vi "Device Panel.vi"(7 "Calling VI Ref":refnum<vi>) -> ()   [LabVIEW 2020]
uses:
  Device Panel Controls/Device Control Information Array.ctl
  Device Panel Controls/Device Control Information.ctl
  <vilib>/Utility/miscctls.llb/LVPointTypeDef.ctl
  Device Manager/Common Device Queue/Common Device Controls/Common Device Actions.ctl
panel:
  in  "Quit All Engines":bool
  in  "Quit":bool
  in  "Devices":T1
  out "Hardware Configuration File Path":path
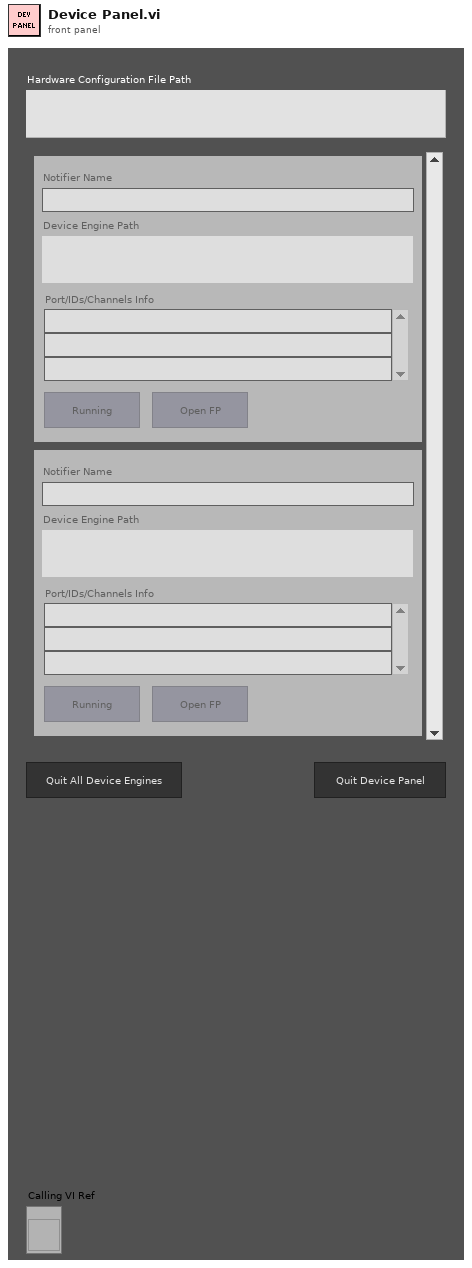
[diagram p1: front panel]
types:
  T1 = typedef "Device Control Information Array.ctl" = T2[]
  T2 = typedef "Device Control Information.ctl" = cluster{"Notifier Name":string, "Device Engine Path":path, "Running?":bool, "Open Front Panel":bool, "Port/IDs/Channels Info":string[]}
  T3 = enum16{"Always On", "Always Off", "Off While Running"}
  T4 = typedef "LVPointTypeDef.ctl" = cluster{"Horizontal":i16, "Vertical":i16}
  T5 = typedef "Common Device Actions.ctl" = enum16{"Specific Action", "Open Front Panel", "Close Front Panel", "Quit", "Quit All"}
  T6 = cluster{"Notifier Name":bool, "Device Engine Path":bool, "Running?":bool, "Open Front Panel":bool, "Port/IDs/Channels Info":bool[]}[]
  T7 = typedef "LVRectTypeDef.ctl" = cluster{"Left":i16, "Top":i16, "Right":i16, "Bottom":i16}
  T8 = typedef "LVBoundsTypeDef.ctl" = cluster{"Width":u32, "Height":u32}
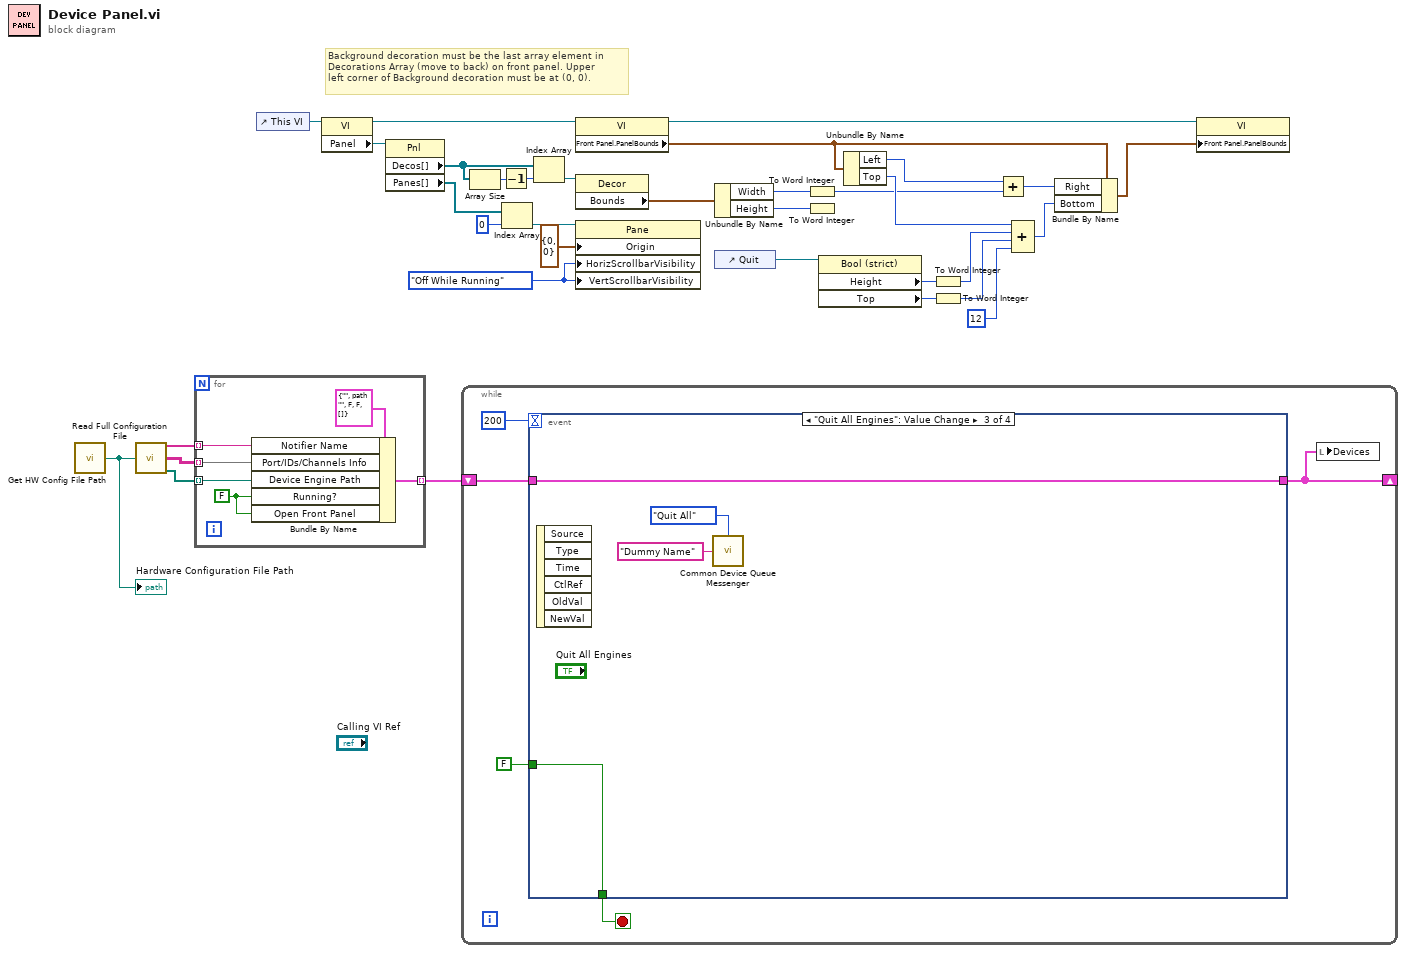
[diagram p0: block diagram]
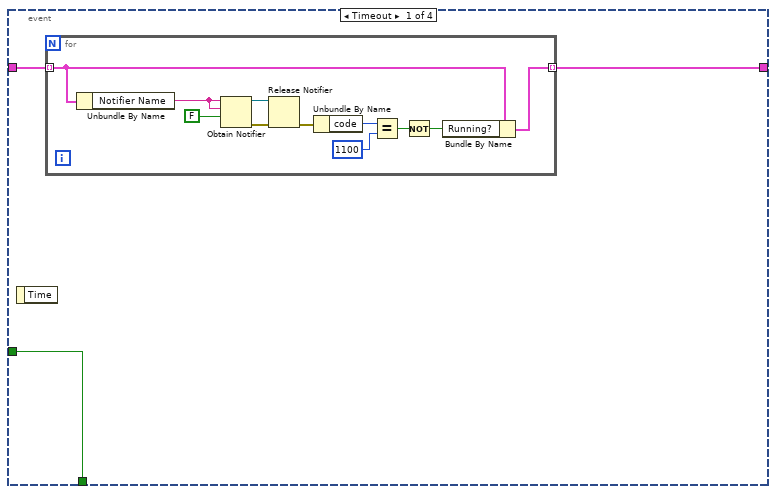
[diagram p2: hidden frame]
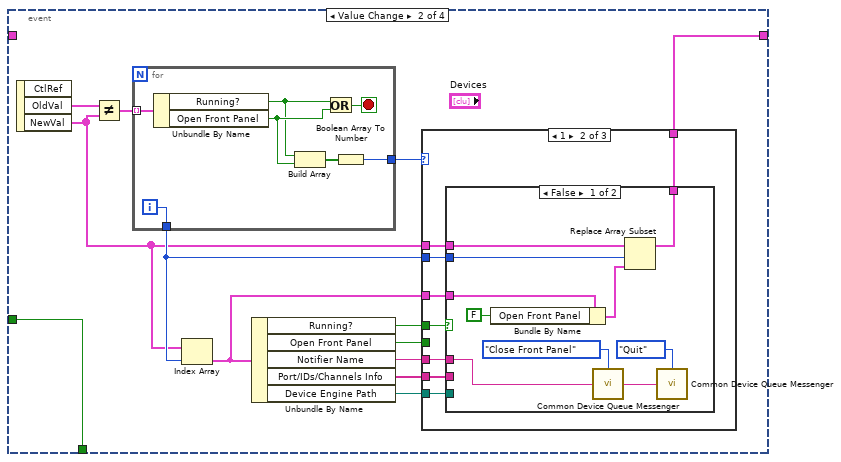
[diagram p3: hidden frame]
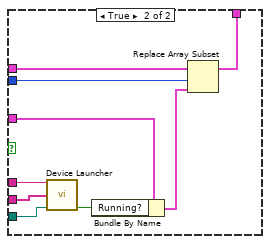
[diagram p5: hidden frame]
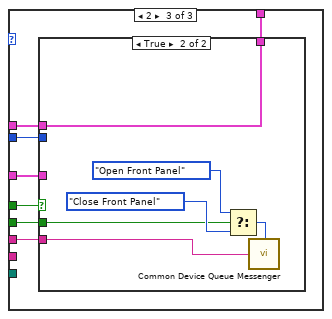
[diagram p6: hidden frame]
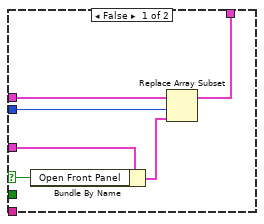
[diagram p7: hidden frame]
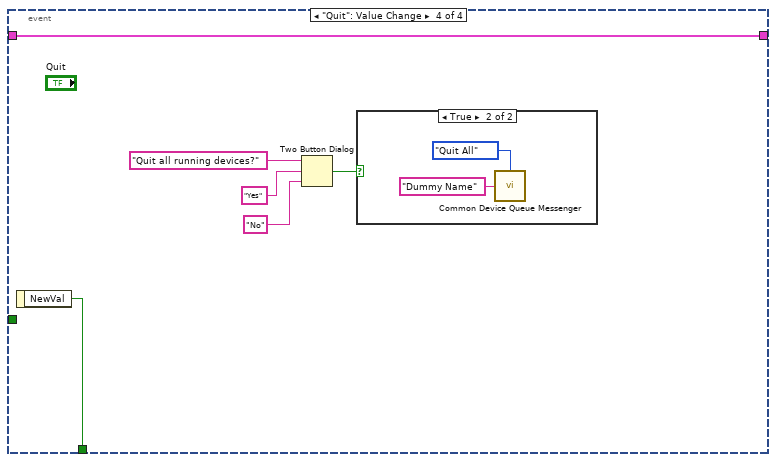
[diagram p8: hidden frame]
diagram:
  w12 = T3."Off While Running" ("Vertical Scrollbar Visibility")
  # "Background decoration must be the last array element in\nDecorations Array (move to back) on front panel. Upper\nleft corner of Background decoration must be at (0, 0)."
  n1 = call "Get HW Config File Path.vi"() -> ("File Path"=w30:path)  [unwired: 14 in, 1 out]
  "Hardware Configuration File Path" <- w30
  n2 = call "Read Full Configuration File.vi"("Config File Path"=w30) -> ("Unique Notifier Names"=w31:string[], "Device Port/ID/Channel Info"=w32:string[][], "Device Engine Paths"=w34:path[])  [unwired: 11 in, 1 out]
  n3 = for {
    tunnel: w34 -> [w39] mode=indexing
    tunnel: [w38] -> w33 mode=indexing
    tunnel: w32 -> [w36] mode=indexing
    tunnel: w31 -> [w35] mode=indexing
    w37 = FALSE ("Open Front Panel")
    n4 = Bundle By Name(cluster=T2 {"Notifier Name"="", "Device Engine Path"=path "", "Running?"=FALSE, "Open Front Panel"=FALSE, "Port/IDs/Channels Info"=[]} ("Device Engine Control"), "Notifier Name"=w35, "Port/IDs/Channels Info"=w36, "Device Engine Path"=w39, "Running?"=w37, "Open Front Panel"=w37) -> (w38:T2)
  }
  n5 = control-ref of="This VI"() -> (w5:refnum<vi>)
  n6 = property class="VI"(reference=w5) -> (reference out=w13:refnum<vi>, "Panel"=w6:refnum<vi>)  [unwired: 1 in, 1 out]
  n7 = property class="Pnl"(reference=w6) -> ("Decos[]"=w4:refnum<vi>[], "Panes[]"=w9:refnum<vi>[])  [unwired: 1 in, 2 out]
  n8 = while {
    shift-right: [w41] -> _
    shift-left: w33 -> [w42]
    stop <- w44 stop-if-true
    n9 = event shown="[2] \"Quit All Engines\": Value Change" {
      selector: _ -> [_ _ _ _]
      dyn-events: _ -> [_ _ _ _]
      timeout: 200 -> [_ _ _ _]
      tunnel: [w48 w72 w130 w136] -> w44
      tunnel: FALSE -> [w48 w72 w130 _]
      tunnel: w42 -> [w47 _ w129 w135]
      tunnel: [w46 w60 w129 w135] -> w41
      event Timeout {
        n10 = event-data() -> ()  [unwired: 1 in, 1 out]
        n11 = for {
          tunnel: w47 -> [w57] mode=indexing
          tunnel: [w56] -> w46 mode=indexing
          n12 = Unbundle By Name(w57) -> ("Notifier Name"=w55:string)
          n13 = Obtain Notifier(name (unnamed)=w55, notification data type=w55, create if not found? (T)=FALSE) -> (notifier out=w50:refnum<notifier>, error out=w51:errorcluster)  [unwired: 1 in, 1 out]
          n14 = Release Notifier(notifier=w50, error in (no error)=w51) -> (error out=w49:errorcluster)  [unwired: 1 in, 2 out]
          n15 = Unbundle By Name(w49) -> ("code"=w59:i32)
          n16 = Equal?(x=w59, y=1100) -> (x = y?=w53:bool)
          n17 = Not(x=w53) -> (.not. x?=w52:bool)
          n18 = Bundle By Name(cluster=w57, "Running?"=w52) -> (w56:T2)
        }
      }
      event Value Change {
        n19 = event-data() -> ("OldVal"=w71:T1, "NewVal"=w62:T1)  [unwired: 1 in, 1 out]
        n20 = Not Equal?(x=w71, y=w62) -> (x != y?=w70:T6)
        n21 = for {
          tunnel: w70 -> [w125] mode=indexing
          tunnel: [w124] -> w63
          tunnel: [w120] -> w69
          i -> [w124]
          stop <- w126 stop-if-true
          n22 = Unbundle By Name(w125) -> ("Running?"=w122:bool, "Open Front Panel"=w123:bool)
          n23 = Build Array(w122, w123) -> (w121:bool[])
          n24 = Or(x=w122, y=w123) -> (x .or. y?=w126:bool)
          n25 = Boolean Array To Number(Boolean array=w121) -> (number=w120:u32)
        }
        n26 = Index Array(array=w62, index=w63) -> (element=w61:T2)
        n27 = Unbundle By Name(w61) -> ("Running?"=w68:bool, "Open Front Panel"=w67:bool, "Notifier Name"=w66:string, "Port/IDs/Channels Info"=w65:string[], "Device Engine Path"=w64:path)
        n28 = case shown="1" w69 {
          tunnel: w68 -> [_ w81 w105]
          tunnel: w67 -> [_ _ w107]
          tunnel: w66 -> [_ w80 w106]
          tunnel: w65 -> [_ w79 _]
          tunnel: w64 -> [_ w78 _]
          tunnel: w62 -> [w73 w77 w104]
          tunnel: w63 -> [_ w76 w101]
          tunnel: w61 -> [_ w75 w102]
          tunnel: [w73 w74 w103] -> w60
          frame Default {
          }
          frame 1 {
            n29 = case shown="False" w81 {
              tunnel: w80 -> [w91 w100]
              tunnel: w79 -> [_ w98]
              tunnel: w78 -> [_ w99]
              tunnel: w77 -> [w85 w97]
              tunnel: w76 -> [w84 w96]
              tunnel: w75 -> [w87 w95]
              tunnel: [w82 w92] -> w74
              frame False {
                n30 = Bundle By Name(cluster=w87, "Open Front Panel"=FALSE) -> (w83:T2)
                n31 = call "Common Device Queue Messenger.vi"("Common Action"=Common_Device_Actions."Close Front Panel" ("Common Actions"), "Notifier Name"=w91) -> ("Notifier Name"=w90:string)  [unwired: 13 in]
                n32 = Replace Array Subset(array=w85, new element=w83, index=w84) -> (w82:T1)
                n33 = call "Common Device Queue Messenger.vi"("Common Action"=Common_Device_Actions."Quit" ("Common Actions"), "Notifier Name"=w90) -> ()  [unwired: 13 in, 1 out]
              }
              frame True {
                n34 = call "Device Launcher.vi"("Notifier Name"=w100, "Device Ports/IDs/Channels"=w98, "Device Engine Path"=w99) -> ("Running?"=w94:bool)  [unwired: 11 in, 1 out]
                n35 = Bundle By Name(cluster=w95, "Running?"=w94) -> (w93:T2)
                n36 = Replace Array Subset(array=w97, new element=w93, index=w96) -> (w92:T1)
              }
            }
          }
          frame 2 {
            n37 = case shown="True" w105 {
              selector: w105 -> [w112 _]
              tunnel: w107 -> [_ w116]
              tunnel: w106 -> [_ w115]
              tunnel: w104 -> [w111 w114]
              tunnel: [w108 w114] -> w103
              tunnel: w102 -> [w113 _]
              tunnel: w101 -> [w110 _]
              frame False {
                n38 = Bundle By Name(cluster=w113, "Open Front Panel"=w112) -> (w109:T2)
                n39 = Replace Array Subset(array=w111, new element=w109, index=w110) -> (w108:T1)
              }
              frame True {
                n40 = Select(t=Common_Device_Actions."Open Front Panel" ("Common Actions"), s=w116, f=Common_Device_Actions."Close Front Panel" ("Common Actions")) -> (s? t:f=w117:T5)
                n41 = call "Common Device Queue Messenger.vi"("Common Action"=w117, "Notifier Name"=w115) -> ()  [unwired: 13 in, 1 out]
              }
            }
          }
        }
      }
      event "Quit All Engines": Value Change {
        n42 = event-data() -> ()  [unwired: 1 in, 6 out]
        n43 = call "Common Device Queue Messenger.vi"("Common Action"=Common_Device_Actions."Quit All" ("Common Actions"), "Notifier Name"="Dummy Name") -> ()  [unwired: 13 in, 1 out]
      }
      event "Quit": Value Change {
        n44 = event-data() -> ("NewVal"=w136:bool)  [unwired: 1 in]
        n45 = Two Button Dialog(message="Quit all running devices?", 1:"No" ("F button name (\"Cancel\")"), 2:"Yes" ("T button name (\"OK\")")) -> (T button?=w131:bool)
        n46 = case shown="True" w131 {
          frame False {
          }
          frame True {
            n47 = call "Common Device Queue Messenger.vi"("Common Action"=Common_Device_Actions."Quit All" ("Common Actions"), "Notifier Name"="Dummy Name") -> ()  [unwired: 13 in, 1 out]
          }
        }
      }
    }
    n48 = local write "Devices"(w41) -> ()
  }
  n49 = Array Size(array=w4) -> (size(s)=w2:i32)
  n50 = Decrement(x=w2) -> (x-1=w3:i32)
  n51 = Index Array(array=w9, index=0) -> (element=w8:refnum<vi>)
  n52 = Index Array(array=w4, index=w3) -> (element=w11:refnum<vi>)
  n53 = property class="VI"(reference=w13) -> (reference out=w15:refnum<vi>, "Front Panel.PanelBounds"=w16:T7)  [unwired: 1 in, 1 out]
  n54 = property class="Decor"(reference=w11) -> ("Bounds"=w14:T8)  [unwired: 1 in, 2 out]
  n55 = property class="Pane"(reference=w8, "Origin"=T4 {"Horizontal"=0, "Vertical"=0}, "HorizScrollbarVisibility"=w12, "VertScrollbarVisibility"=w12) -> ()  [unwired: 1 in, 2 out]
  n56 = Unbundle By Name(w14) -> ("Width"=w19:u32, "Height"=w22:u32)
  n57 = control-ref of="Quit"() -> (w1:refnum<vi>)
  n58 = To Word Integer(number=w19) -> (16bit integer=w21:i16)
  n59 = To Word Integer(number=w22) -> ()  [unwired: 1 out]
  n60 = property class="Bool (strict)"(reference=w1) -> ("Height"=w24:u32, "Top"=w25:i32)  [unwired: 1 in, 2 out]
  n61 = Unbundle By Name(w16) -> ("Left"=w18:i16, "Top"=w29:i16)
  n62 = To Word Integer(number=w24) -> (16bit integer=w27:i16)
  n63 = To Word Integer(number=w25) -> (16bit integer=w28:i16)
  n64 = Add(x=w18, y=w21) -> (x+y=w20:i16)
  n65 = Compound Arithmetic op=ADD(w29, w27, w28, i16 12 ("y")) -> (w23:i16)
  n66 = Bundle By Name(cluster=w16, "Right"=w20, "Bottom"=w23) -> (w17:T7)
  n67 = property class="VI"(reference=w15, "Front Panel.PanelBounds"=w17) -> ()  [unwired: 1 in, 2 out]
